vi "enterDriveMode.vi"(8 "error in (no error)":errorcluster, 9 "targetNumber":i16, 10 "interface object in":refnum<k20>, 11 "MotorController in":refnum<class "MotorController.lvclass">) -> (0 "error out":errorcluster, 2 "interface object out":refnum<k20>, 3 "MotorController out":refnum<class "MotorController.lvclass">, 4 "targetTorqueRes":u32, 5 "controlWord6Res":i16)   [LabVIEW 2018, in "MotorController.lvclass"]
uses:
  MotorController.lvclass
  MotorController.lvclass/MotorController.ctl
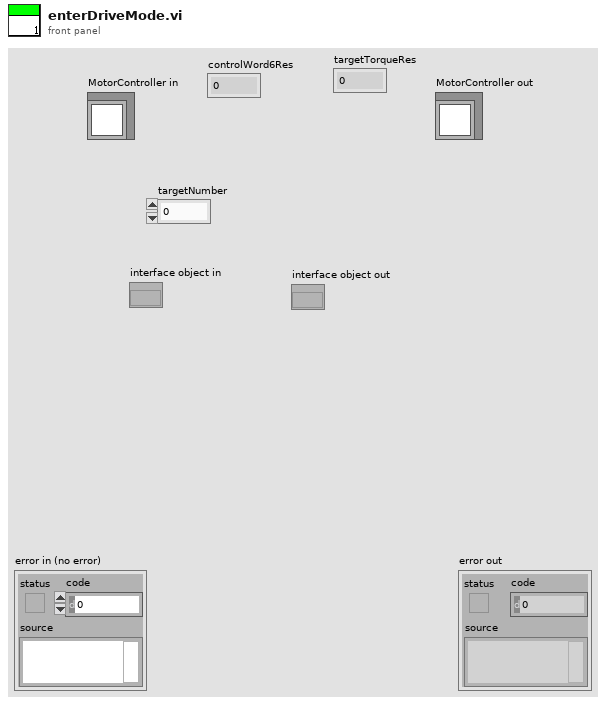
[diagram p1: front panel]
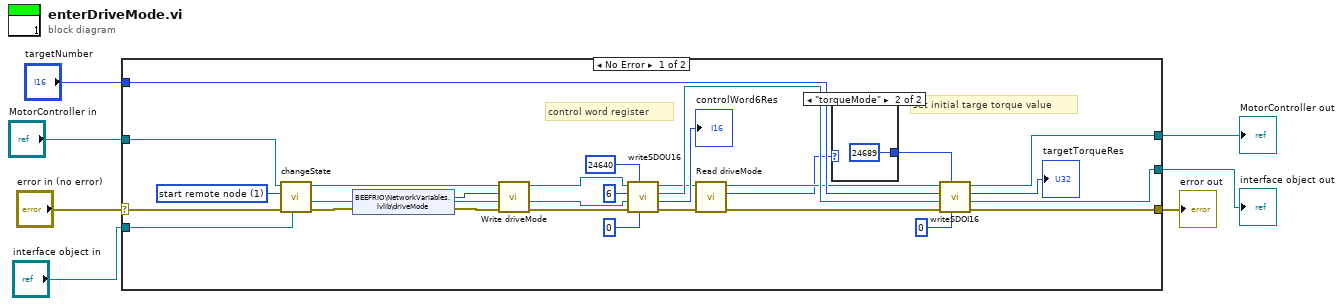
[diagram p0: block diagram]
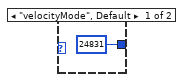
[diagram p2: hidden frame]
diagram:
  n1 = case shown="No Error" "error in (no error)" {
    selector: "error in (no error)" -> [w33 w39]
    tunnel: [w23 w39] -> w6
    tunnel: [w22 w38] -> w4
    tunnel: "MotorController in" -> [w31 w38]
    tunnel: "interface object in" -> [w30 _]
    tunnel: "targetNumber" -> [w25 _]
    tunnel: [w20 _] -> w1
    frame No Error {
      w32 = u16 1 items=["start remote node"=1, "stop remote node"=2, "enter pre-operational"=128, "reset node"=129, "reset communication"=130] ("state")
      # "set initial targe torque value"
      # "control word register"
      n2 = call "changeState.vi"("interface object in"=w30, "error in (no error)"=w33, "state"=w32, "MotorController in"=w31) -> ("error out"=w9:errorcluster, "interface object out"=w29:refnum<k20>, "MotorController out"=w11:refnum<class "MotorController.lvclass">)  [unwired: 5 in]
      n3 = shared-variable "BEEFRIO\\NetworkVariables.lvlib\\driveMode"(error in=w9) -> (w10:enum16{"velocityMode", "torqueMode", ""}, error out=w8:errorcluster)
      n4 = call "Write driveMode.vi"("error in (no error)"=w8, "driveMode"=w10, "MotorController in"=w11) -> ("error out"=w12:errorcluster, "MotorController out"=w13:refnum<class "MotorController.lvclass">)  [unwired: 7 in]
      n5 = call "writeSDOU16.vi"("object sub-index (0)"=u8 0, "object index"=u16 24640, "error in (no error)"=w12, "interface object in"=w29, "inputNumber"=u16 6, "MotorController in"=w13) -> ("error out"=w18:errorcluster, "completion code"=→"controlWord6Res":u32, "interface object out"=w26:refnum<k20>, "MotorController out"=w19:refnum<class "MotorController.lvclass">)  [unwired: 2 in]
      n6 = call "Read driveMode.vi"("error in (no error)"=w18, "MotorController in"=w19) -> ("error out"=w15:errorcluster, "driveMode"=w16:enum16{"velocityMode", "torqueMode", ""}, "MotorController out"=w17:refnum<class "MotorController.lvclass">)  [unwired: 7 in]
      n7 = case shown="\"torqueMode\"" w16 {
        tunnel: [u16 24831 ("object index") u16 24689 ("object index")] -> w14
        frame "velocityMode", Default {
        }
        frame "torqueMode" {
        }
      }
      n8 = call "writeSDOI16.vi"("object sub-index (0)"=u8 0, "object index"=w14, "error in (no error)"=w15, "interface object in"=w26, "inputNumber"=w25, "MotorController in"=w17) -> ("error out"=w23:errorcluster, "interface object out"=w20:refnum<k20>, "completion code"=→"targetTorqueRes":u32, "MotorController out"=w22:refnum<class "MotorController.lvclass">)  [unwired: 2 in]
    }
    frame Error {
    }
  }
  "error out" <- w6
  "MotorController out" <- w4
  "interface object out" <- w1
